vi "Program ILC.vi"(0 "Model in":refnum<class "Model.lvclass">, 11 "error in (no error)":errorcluster) -> (4 "Model out":refnum<class "Model.lvclass">, 15 "error out":errorcluster)   [LabVIEW 2016, in "Model.lvclass"]
uses:
  Model.lvclass
  Model.lvclass/Model.ctl
  Modbus/DesktopModbus/DesktopModbus.lvclass
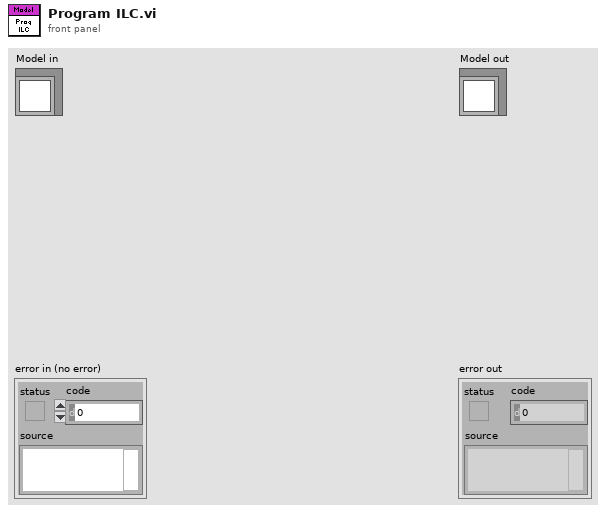
[diagram p1: front panel]
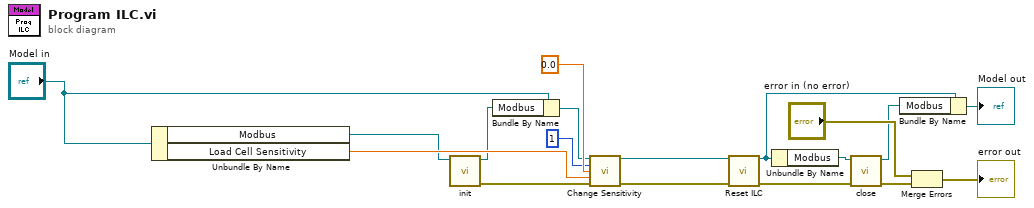
[diagram p0: block diagram]
diagram:
  n1 = Unbundle By Name("Model in") -> ("Modbus"=w15:refnum<class "DesktopModbus.lvclass">, "Load Cell Sensitivity"=w17:dbl)
  n2 = call "init.vi"("DesktopModbus in"=w15) -> ("error out"=w5:errorcluster, "DesktopModbus out"=w11:refnum<class "DesktopModbus.lvclass">)  [unwired: 9 in]
  n3 = Bundle By Name(cluster="Model in", "Modbus"=w11) -> (w6:refnum<class "Model.lvclass">)
  n4 = call "Change Sensitivity.vi"("Model in"=w6, "Channel"=u8 1, "Offset"=sgl 0.0, "Sensitivity"=w17, "error in (no error)"=w5) -> ("Model out"=w2:refnum<class "Model.lvclass">, "error out"=w1:errorcluster)  [unwired: 9 in]
  n5 = call "Reset ILC.vi"("Model in"=w2, "error in (no error)"=w1) -> ("Model out"=w4:refnum<class "Model.lvclass">, "error out"=w3:errorcluster)  [unwired: 12 in]
  n6 = Unbundle By Name(w4) -> ("Modbus"=w10:refnum<class "DesktopModbus.lvclass">)
  n7 = call "close.vi"("error in (no error)"=w3, "DesktopModbus in"=w10) -> ("error out"=w7:errorcluster, "DesktopModbus out"=w9:refnum<class "DesktopModbus.lvclass">)  [unwired: 8 in]
  n8 = Bundle By Name(cluster=w4, "Modbus"=w9) -> (→"Model out":refnum<class "Model.lvclass">)
  n9 = Merge Errors("error in (no error)", w7) -> (→"error out":errorcluster)
